vi "Run SQL.vi"(8 "error in (no error)":errorcluster, 10 "SQL":string, 11 "Data Manager in":refnum<class "Data Manager.lvclass">) -> (0 "error out":errorcluster, 1 "Result Set":string[][](table) caption="Result Set (from first statement with results)", 2 "Column Names":string[](array[string]), 3 "Data Manager out":refnum<class "Data Manager.lvclass">)   [LabVIEW 2020, in "Data Manager.lvclass"]
uses:
  Data Manager.lvclass
  Data Manager.lvclass/Data Manager.ctl
  <vilib>/drjdpowell/SQLite Library/SQL Connection/Execute SQL.vi
  <vilib>/drjdpowell/SQLite Library/SQLite.lvlib
  <vilib>/drjdpowell/SQLite Library/SQL Connection/Connection.lvclass
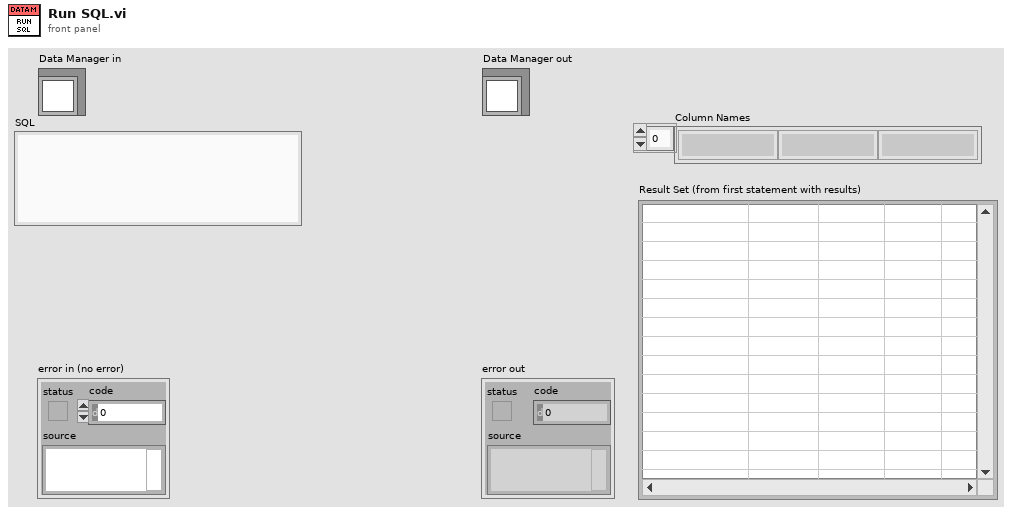
[diagram p1: front panel]
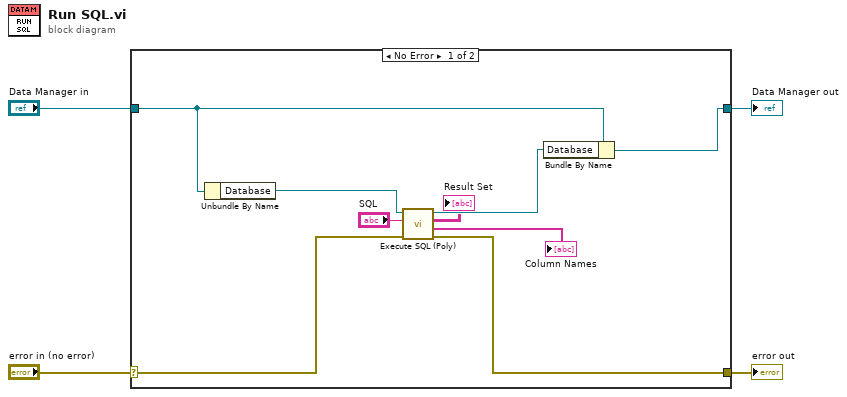
[diagram p0: block diagram]
diagram:
  n1 = case shown="No Error" "error in (no error)" {
    selector: "error in (no error)" -> [w5 w15]
    tunnel: [w6 w15] -> w3
    tunnel: [w12 w14] -> w1
    tunnel: "Data Manager in" -> [w13 w14]
    frame No Error {
      n2 = Unbundle By Name(w13) -> ("Database"=w10:refnum<class "Connection.lvclass">)
      n3 = call-poly <vilib>:"Execute SQL (Poly).vi"("error in (no error)"=w5, "SQL"="SQL", "SQLite Connection in"=w10) -> ("error out"=w6:errorcluster, "Column Names"=→"Column Names":string[], "Result Set"=→"Result Set":string[][], "SQLite Connection"=w11:refnum<class "Connection.lvclass">)  [unwired: 5 in]
      n4 = Bundle By Name(cluster=w13, "Database"=w11) -> (w12:refnum<class "Data Manager.lvclass">)
    }
    frame Error {
    }
  }
  "error out" <- w3
  "Data Manager out" <- w1
